vi "Export Experiment Data.vi"(9 "Skip Export":bool, 10 "Export?":bool, 11 "Data":dbl[][](array[numeric])) -> (3 "Export Complete?":bool)   [LabVIEW 2016]
uses:
  <vilib>/Utility/error.llb/DialogType.ctl
  <vilib>/Utility/file.llb/Write Delimited Spreadsheet (string).vi
  <vilib>/Utility/file.llb/Write Delimited Spreadsheet (DBL).vi
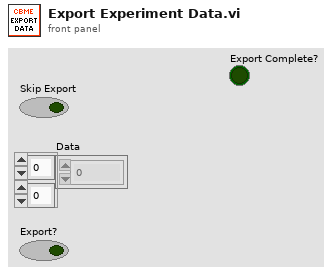
[diagram p1: front panel]
types:
  T1 = enum16{"open", "replace", "create", "open or create", "replace or create", "replace or create with confirmation"}
  T2 = typedef "DialogType.ctl" = u16
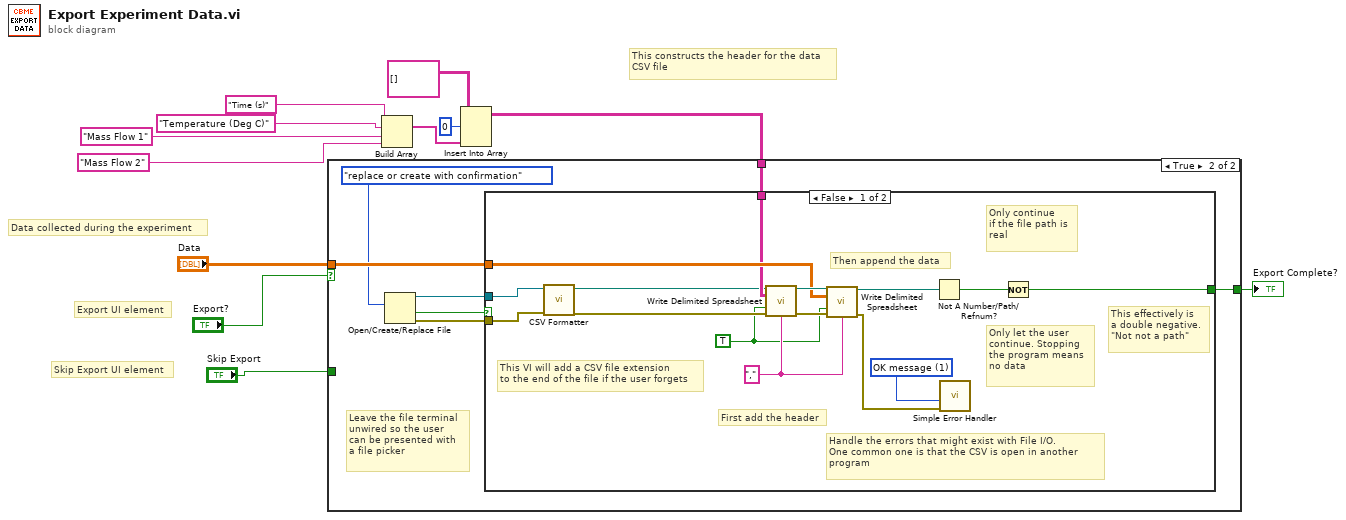
[diagram p0: block diagram]
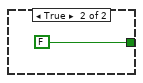
[diagram p3: hidden frame]
diagram:
  # "Skip Export UI element"
  # "Export UI element"
  # "Data collected during the experiment"
  # "This constructs the header for the data\nCSV file"
  n1 = Build Array("Time (s)", "Temperature (Deg C)", "Mass Flow 1", "Mass Flow 2") -> (w7:string[])
  n2 = Insert Into Array(array=string[][] [], index (row)=0, new element=w7) -> (w10:string[][])  [unwired: 1 in]
  n3 = case shown="True" "Export?" {
    tunnel: "Data" -> [_ w19]
    tunnel: [w13 w20] -> w4
    tunnel: "Skip Export" -> [w13 _]
    tunnel: w10 -> [_ w18]
    frame False {
      # "The user doesn't want to export,\nso skip this step"
    }
    frame True {
      # "Leave the file terminal \nunwired so the user \ncan be presented with \na file picker"
      n4 = Open/Create/Replace File(operation (0:open)=T1."replace or create with confirmation") -> (refnum out=w14:refnum<file>, cancelled=w16:bool, error out=w15:errorcluster)  [unwired: 5 in]
      n5 = case shown="False" w16 {
        tunnel: [w33 FALSE] -> w20
        tunnel: w19 -> [w30 _]
        tunnel: w18 -> [w29 _]
        tunnel: w15 -> [w25 _]
        tunnel: w14 -> [w24 _]
        frame False {
          w26 = T2 1 items=["no dialog", "OK message", "continue or stop message", "OK message + warnings", "continue/stop + warnings"] ("type of dialog (OK msg:1)")
          w22 = TRUE ("append to file? (new file:F)")
          w28 = "," ("delimiter (\\t)")
          # "This VI will add a CSV file extension\nto the end of the file if the user forgets"
          # "Only let the user\ncontinue. Stopping\nthe program means\nno data"
          # "Handle the errors that might exist with File I/O.\nOne common one is that the CSV is open in another\nprogram"
          # "This effectively is\na double negative.\n\"Not not a path\""
          # "Only continue\nif the file path is \nreal"
          # "Then append the data"
          # "First add the header"
          n6 = call "CSV Formatter.vi"("error in (no error)"=w25, "Byte Stream File in"=w24) -> ("error out"=w23:errorcluster, "path"=w21:path)  [unwired: 8 in]
          n7 = call-poly <vilib>:"Write Delimited Spreadsheet.vi"("file path (dialog if empty)"=w21, "2D data"=w29, "append to file? (new file:F)"=w22, "error in (no error)"=w23, "delimiter (\\t)"=w28) -> ("new file path (Not A Path if cancelled)"=w32:path, "error out"=w31:errorcluster)  [unwired: 9 in]
          n8 = call-poly <vilib>:"Write Delimited Spreadsheet.vi"("file path (dialog if empty)"=w32, "2D data"=w30, "append to file? (new file:F)"=w22, "error in (no error)"=w31, "delimiter (\\t)"=w28) -> ("new file path (Not A Path if cancelled)"=w35:path, "error out"=w27:errorcluster)  [unwired: 9 in]
          n9 = Not A Number/Path/Refnum?(number/path/refnum=w35) -> (NaN/Path/Refnum?=w34:bool)
          n10 = call <vilib>:"Simple Error Handler.vi"("type of dialog (OK msg:1)"=w26, "error in (no error)"=w27) -> ()  [unwired: 3 in, 5 out]
          n11 = Not(x=w34) -> (.not. x?=w33:bool)
        }
        frame True {
        }
      }
    }
  }
  "Export Complete?" <- w4
